vi "turret_raw_to_degrees.vi"(10 "Raw Encoder Units In":i32) -> (2 "Degrees Out":dbl)   [LabVIEW 2020]
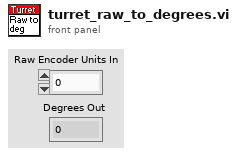
[diagram p1: front panel]
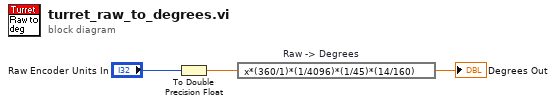
[diagram p0: block diagram]
diagram:
  n1 = To Double Precision Float(number="Raw Encoder Units In") -> (double precision float=w1:dbl)
  n2 = expression code="x*(360/1)*(1/4096)*(1/45)*(14/160)" "Raw -> Degrees"(w1) -> (→"Degrees Out":dbl)
